vi "ExtractRecords.vi"(6 "Buffer mode":T1, 8 "5782 records":u16[](array[numeric]), 9 "5160 records":i32[](array[numeric]), 10 "5782 Data":u64[](array[numeric]), 11 "5160 Data":u64[](array[numeric])) -> (2 "5782 Data out":u64[](array[numeric]), 3 "5160 Data out":u64[](array[numeric]))   [LabVIEW 2013]
uses:
  controls/Data_display_mode.ctl
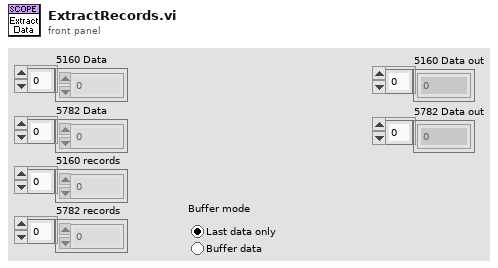
[diagram p1: front panel]
types:
  T1 = typedef "Data_display_mode.ctl" = enum32{"Last data only", "Buffer data"}
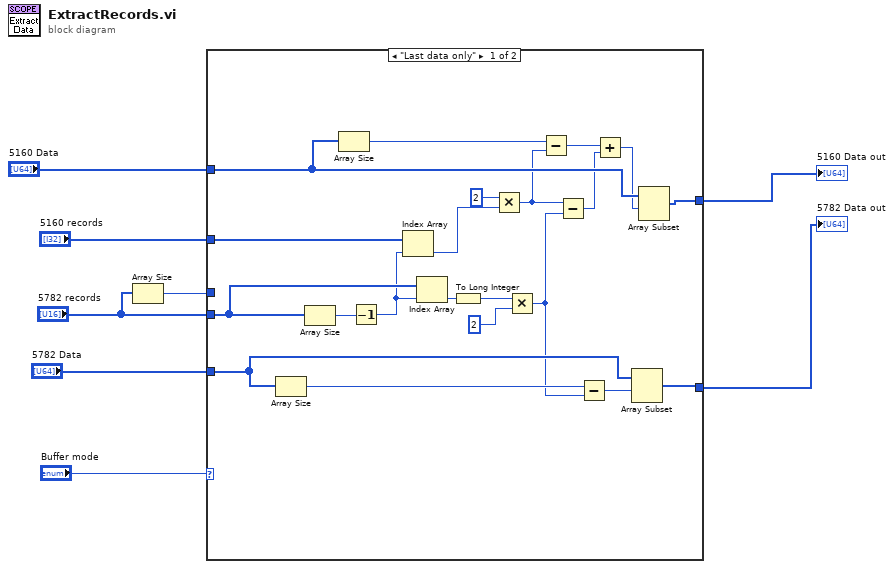
[diagram p0: block diagram]
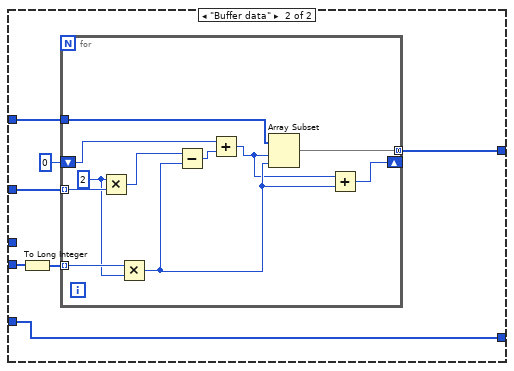
[diagram p2: hidden frame]
diagram:
  n1 = Array Size(array="5782 records") -> (size(s)=w1:i32)
  n2 = case shown="\"Last data only\"" "Buffer mode" {
    tunnel: "5782 records" -> [w28 w34]
    tunnel: "5160 records" -> [w21 w36]
    tunnel: "5782 Data" -> [w24 w31]
    tunnel: [w23 w31] -> w4
    tunnel: "5160 Data" -> [w14 w35]
    tunnel: [w20 w30] -> w5
    tunnel: w1 -> [_ _]
    frame "Last data only" {
      n3 = Array Size(array=w24) -> (size(s)=w22:i32)
      n4 = Array Size(array=w28) -> (size(s)=w29:i32)
      n5 = Array Size(array=w14) -> (size(s)=w13:i32)
      n6 = Decrement(x=w29) -> (x-1=w27:i32)
      n7 = Index Array(array=w21, index=w27) -> (element=w16:i32)
      n8 = Index Array(array=w28, index=w27) -> (element=w19:u16)
      n9 = To Long Integer(number=w19) -> (32bit integer=w18:i32)
      n10 = Multiply(x=2, y=w16) -> (x*y=w12:i32)
      n11 = Multiply(x=w18, y=2) -> (x*y=w17:i32)
      n12 = Subtract(x=w13, y=w12) -> (x-y=w11:i32)
      n13 = Subtract(x=w12, y=w17) -> (x-y=w10:i32)
      n14 = Subtract(x=w22, y=w17) -> (x-y=w25:i32)
      n15 = Add(x=w11, y=w10) -> (x+y=w9:i32)
      n16 = Array Subset(array=w24, index=w25) -> (w23:u64[])  [unwired: 1 in]
      n17 = Array Subset(array=w14, index=w9) -> (w20:u64[])  [unwired: 1 in]
    }
    frame "Buffer data" {
      n18 = To Long Integer(number=w34) -> (32bit integer=w33:i32[])
      n19 = for {
        tunnel: w36 -> [w44] mode=indexing
        tunnel: w35 -> [w47]
        tunnel: [w46] -> w30 mode=concatenating
        tunnel: w33 -> [w43] mode=indexing
        shift-right: [w40] -> _
        shift-left: 0 -> [w39]
        w42 = 2 ("x")
        n20 = Multiply(x=w42, y=w44) -> (x*y=w45:i32)
        n21 = Multiply(x=w43, y=w42) -> (x*y=w41:i32)
        n22 = Subtract(x=w45, y=w41) -> (x-y=w38:i32)
        n23 = Add(x=w39, y=w38) -> (x+y=w37:i32)
        n24 = Array Subset(array=w47, index=w37, length=w41) -> (w46:u64[])
        n25 = Add(x=w37, y=w41) -> (x+y=w40:i32)
      }
    }
  }
  "5160 Data out" <- w5
  "5782 Data out" <- w4
